vi "Renew Splitter Height.vi"(8 "error in (no error)":errorcluster, 9 "Pane Ref":refnum<vi>, 10 "Splitter Ref":refnum<vi>, 11 "ScriptDialog.lvclass":refnum<class "ScriptDialog.lvclass">) -> (0 "error out":errorcluster, 3 "ScriptDialog.lvclass Out":refnum<class "ScriptDialog.lvclass">)   [LabVIEW 2015, in "ScriptDialog.lvclass"]
uses:
  ScriptDialog.lvclass
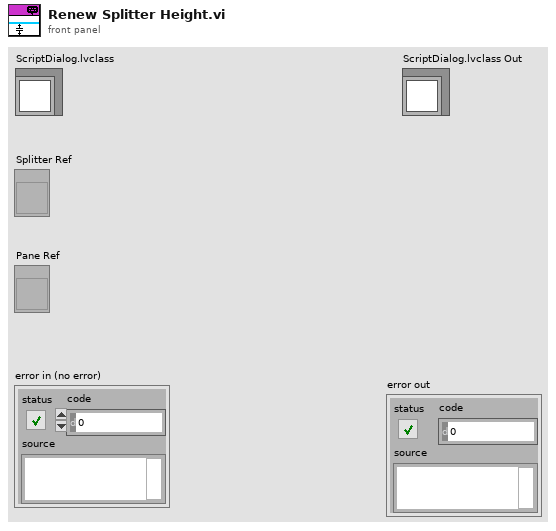
[diagram p1: front panel]
types:
  T1 = typedef "LVBoundsTypeDef.ctl" = cluster{"Width":u32, "Height":u32}
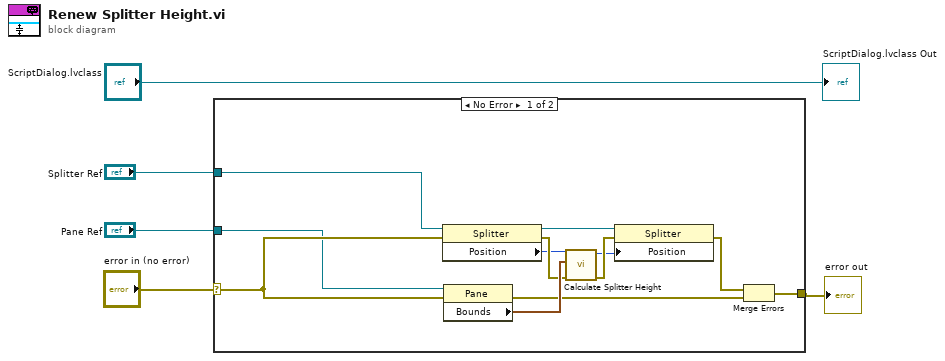
[diagram p0: block diagram]
diagram:
  n1 = case shown="No Error" "error in (no error)" {
    selector: "error in (no error)" -> [w13 w18]
    tunnel: [w8 w18] -> w3
    tunnel: "Splitter Ref" -> [w7 _]
    tunnel: "Pane Ref" -> [w6 _]
    frame No Error {
      n2 = property class="Splitter"(reference=w7, error in=w13) -> (reference out=w14:refnum<vi>, error out=w12:errorcluster, "Position"=w11:i32)
      n3 = property class="Pane"(reference=w6, error in=w13) -> (error out=w9:errorcluster, "Bounds"=w17:T1)  [unwired: 1 out]
      n4 = call "Calculate Splitter Height.vi"("error in (no error)"=w12, "Panel Bounds"=w17, "Splitter Height"=w11) -> ("error out"=w16:errorcluster, "Splitter Height"=w15:i32)  [unwired: 7 in]
      n5 = property class="Splitter"(reference=w14, error in=w16, "Position"=w15) -> (error out=w10:errorcluster)  [unwired: 1 out]
      n6 = Merge Errors(w10, w9) -> (w8:errorcluster)
    }
    frame Error {
    }
  }
  "error out" <- w3
  "ScriptDialog.lvclass Out" <- "ScriptDialog.lvclass"
